vi "AES - Decrypt String.vi"(8 "error in (no error)":errorcluster, 9 "IV":u8[](array[numeric]), 10 "key":u8[](array[numeric]), 11 "encrypted string":string) -> (0 "error out":errorcluster, 3 "decrypted string":string)   [LabVIEW 2013]
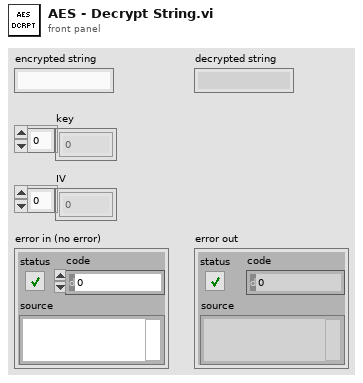
[diagram p1: front panel]
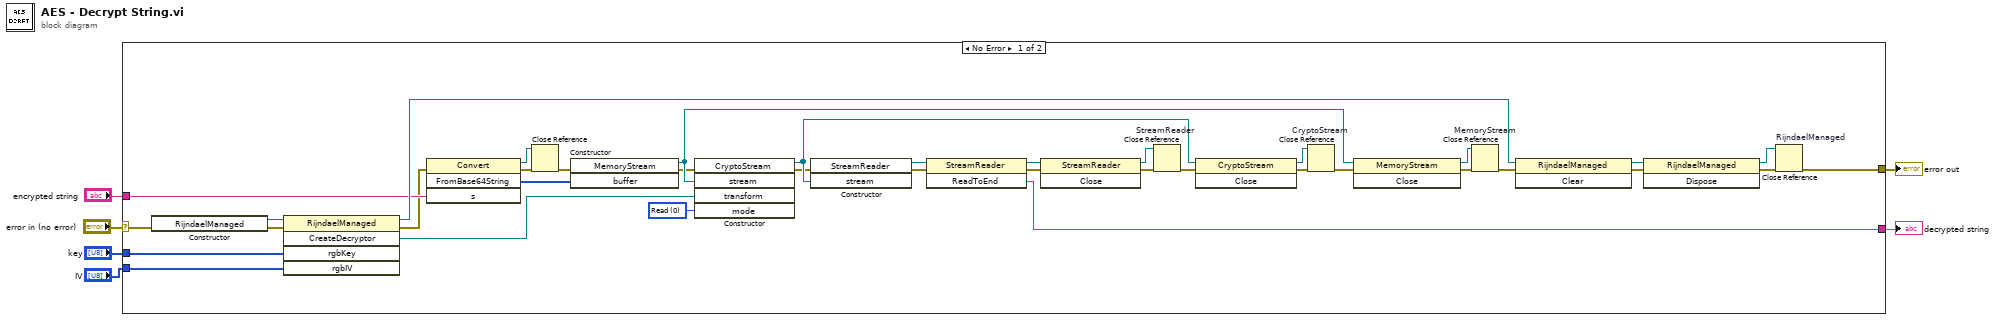
[diagram p0: block diagram]
diagram:
  n1 = case shown="No Error" "error in (no error)" {
    selector: "error in (no error)" -> [w16 w44]
    tunnel: "IV" -> [w25 _]
    tunnel: "key" -> [w24 _]
    tunnel: [w15 w44] -> w3
    tunnel: "encrypted string" -> [w13 _]
    tunnel: [w11 _] -> w1
    frame No Error {
      w19 = 0 items=["Read", "Write"] ("mode")
      n2 = constructor class="RijndaelManaged"(error in=w16) -> (reference out=w21:refnum<k24>, error out=w20:errorcluster)  [unwired: 2 in, 1 out]
      n3 = invoke class="RijndaelManaged" method="CreateDecryptor"(reference=w21, error in=w20, "rgbKey"=w24, "rgbIV"=w25) -> (reference out=w37:refnum<k24>, error out=w7:errorcluster, "CreateDecryptor"=w18:refnum<k24>)  [unwired: 1 in, 2 out]
      n4 = invoke class="Convert" method="FromBase64String"(error in=w7, "s"=w13) -> (reference out=w9:refnum<k24>, error out=w10:errorcluster, "FromBase64String"=w12:u8[])  [unwired: 2 in, 1 out]
      n5 = Close Reference(reference=w9, error in (no error)=w10) -> (error out=w8:errorcluster)
      n6 = constructor class="MemoryStream"(error in=w8, "buffer"=w12) -> (reference out=w30:refnum<k24>, error out=w17:errorcluster)  [unwired: 2 in, 2 out]
      n7 = constructor class="CryptoStream"(error in=w17, "stream"=w30, "transform"=w18, "mode"=w19) -> (reference out=w28:refnum<k24>, error out=w22:errorcluster)  [unwired: 2 in, 4 out]
      n8 = constructor class="StreamReader"(error in=w22, "stream"=w28) -> (reference out=w14:refnum<k24>, error out=w23:errorcluster)  [unwired: 2 in, 2 out]
      n9 = invoke class="StreamReader" method="ReadToEnd"(reference=w14, error in=w23) -> (reference out=w26:refnum<k24>, error out=w27:errorcluster, "ReadToEnd"=w11:string)  [unwired: 1 in]
      n10 = invoke class="StreamReader" method="Close"(reference=w26, error in=w27) -> (reference out=w32:refnum<k24>, error out=w29:errorcluster)  [unwired: 1 in, 1 out]
      n11 = Close Reference "StreamReader"(reference=w32, error in (no error)=w29) -> (error out=w31:errorcluster)
      n12 = invoke class="CryptoStream" method="Close"(reference=w28, error in=w31) -> (reference out=w34:refnum<k24>, error out=w33:errorcluster)  [unwired: 1 in, 1 out]
      n13 = Close Reference "CryptoStream"(reference=w34, error in (no error)=w33) -> (error out=w43:errorcluster)
      n14 = invoke class="MemoryStream" method="Close"(reference=w30, error in=w43) -> (reference out=w36:refnum<k24>, error out=w35:errorcluster)  [unwired: 1 in, 1 out]
      n15 = Close Reference "MemoryStream"(reference=w36, error in (no error)=w35) -> (error out=w40:errorcluster)
      n16 = invoke class="RijndaelManaged" method="Clear"(reference=w37, error in=w40) -> (reference out=w39:refnum<k24>, error out=w38:errorcluster)  [unwired: 1 in, 1 out]
      n17 = invoke class="RijndaelManaged" method="Dispose"(reference=w39, error in=w38) -> (reference out=w42:refnum<k24>, error out=w41:errorcluster)  [unwired: 1 in, 1 out]
      n18 = Close Reference "RijndaelManaged"(reference=w42, error in (no error)=w41) -> (error out=w15:errorcluster)
    }
    frame Error {
    }
  }
  "error out" <- w3
  "decrypted string" <- w1
